vi "Escribir.vi"() -> ()   [LabVIEW 2019]
panel:
  in  "stop":bool
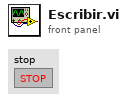
[diagram p1: front panel]
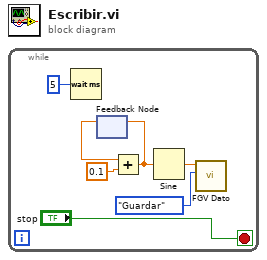
[diagram p0: block diagram]
diagram:
  n1 = while {
    stop <- "stop" stop-if-true
    n2 = Wait (ms)(milliseconds to wait=u32 5) -> ()  [unwired: 1 out]
    n3 = feedback #1() -> (w7:dbl)  [unwired: 1 in]
    n4 = Add(x=w7, y=0.1) -> (x+y=w6:dbl)
    n5 = feedback-in #1(w6) -> ()
    n6 = Sine(x=w6) -> (sin(x)=w4:dbl)
    n7 = call "FGV Dato.vi"("Funcion"=enum16{"Guardar", "Leer"}."Guardar", "Dato In"=w4) -> ()  [unwired: 9 in, 1 out]
  }
